vi "Configure Event Search (Serial Bus - LIN - Symbolic).vi"(7 "Search Value (1)":dbl=1.0, 8 "error in (no error)":errorcluster, 9 "Search Signal ()":string, 10 "Search Message  ()":string, 11 "VISA resource name":refnum<visa-resource-name>) -> (0 "error out":errorcluster, 3 "VISA resource name out":refnum<visa-resource-name>)   [LabVIEW 2023, in "Keysight-DSQx3014T.lvlib"]
doc: "Configures the event search symbolic of LIN bus. Used when the Search Operation is Symbolic Frame, or Symbolic Frame and Signal Value is set in <b>Configure Event Serarch (Serial Bus-Lin)</b>.\n\n<b>Note:</b>\nBefore this VI is called LIN symbolic data (a .ldf file) must be loaded into the oscilloscope using <b>Recall Data From File </b>.vi. A serial bus must be configured for LIN-Symbolic decode and the lister for that serial bus must be enabled (visible on the screen) before calling this VI."
uses:
  Keysight-DSQx3014T.lvlib
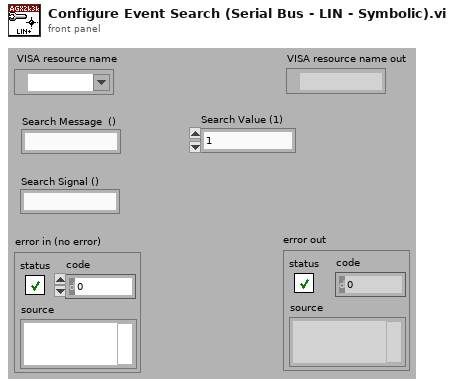
[diagram p1: front panel]
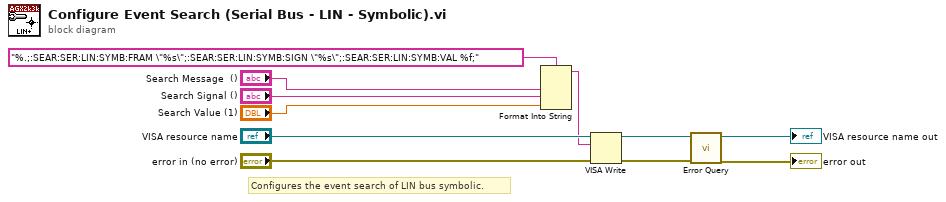
[diagram p0: block diagram]
diagram:
  # "Configures the event search of LIN bus symbolic."
  n1 = Format Into String(format string="%.;:SEAR:SER:LIN:SYMB:FRAM \"%s\";:SEAR:SER:LIN:SYMB:SIGN \"%s\";:SEAR:SER:LIN:SYMB:VAL %f;", "Search Message  ()", "Search Signal ()", "Search Value (1)") -> (resulting string=w1:string)  [unwired: 2 in, 1 out]
  n2 = VISA Write(VISA resource name="VISA resource name", write buffer=w1, error in (no error)="error in (no error)") -> (VISA resource name out=w9:refnum<visa-resource-name>, error out=w8:errorcluster)  [unwired: 1 out]
  n3 = call "Error Query.vi"("error in (no error)"=w8, "VISA resource name"=w9) -> ("error out"=→"error out":errorcluster, "VISA resource name out"=→"VISA resource name out":refnum<visa-resource-name>)  [unwired: 8 out]
